vi "Decimate Linear XY.vi"(6 "Width":u32, 8 "error in (no error)":errorcluster, 9 "Xmin":dbl, 10 "Xmax":dbl, 11 "Data to Decimate":cluster{"X":dbl[], "Y":dbl[]}[](array[cluster])) -> (0 "error out":errorcluster, 3 "Decimated Data":cluster{"X":dbl[], "Y":dbl[]}[](array[cluster]))   [LabVIEW 2022 SP3, in "Decimation.lvlib"]
doc: "Decimate XY array to optimize the density of points per pixel to 2 : Min & Max per pixel."
uses:
  Decimation.lvlib
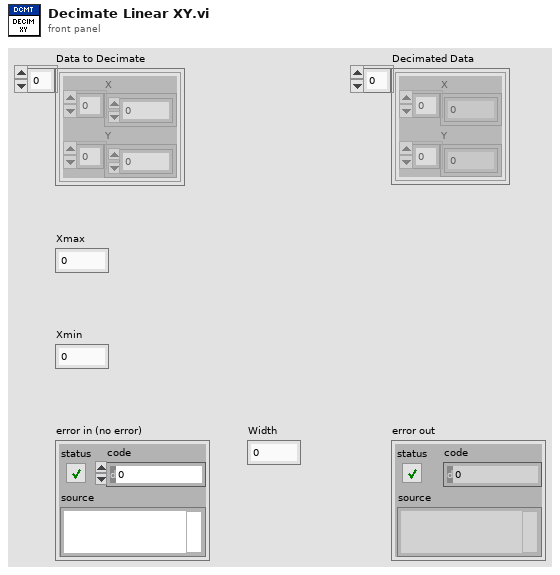
[diagram p1: front panel]
types:
  T1 = cluster{"Decimated Data":dbl[], "Decimated Data":dbl[]}
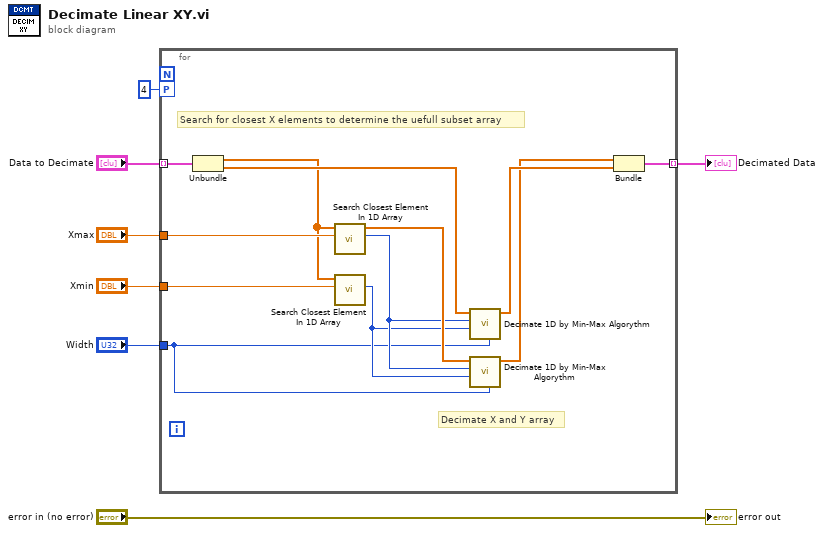
[diagram p0: block diagram]
diagram:
  n1 = for {
    tunnel: "Data to Decimate" -> [w18] mode=indexing
    tunnel: "Xmin" -> [w17]
    tunnel: "Xmax" -> [w16]
    tunnel: [w15] -> w3 mode=indexing
    workers-P: 4 -> [_]
    tunnel: "Width" -> [w10]
    # "Decimate X and Y array"
    # "Search for closest X elements to determine the uefull subset array"
    n2 = Unbundle(w18) -> ("X"=w13:dbl[], "Y"=w14:dbl[])
    n3 = call "Search Closest Element In 1D Array.vi"("Desired element"=w16, "1D Array"=w13) -> ("Closest Index"=w12:i32)  [unwired: 8 in, 1 out]
    n4 = call "Search Closest Element In 1D Array.vi"("Desired element"=w17, "1D Array"=w13) -> ("Closest Index"=w11:i32)  [unwired: 8 in, 1 out]
    n5 = call "Decimate 1D by Min-Max Algorythm.vi"("Width"=w10, "Min Index"=w11, "Max Index"=w12, "Data To Decimate"=w14) -> ("Decimated Data"=w9:dbl[])  [unwired: 6 in, 1 out]
    n6 = call "Decimate 1D by Min-Max Algorythm.vi"("Width"=w10, "Min Index"=w11, "Max Index"=w12, "Data To Decimate"=w13) -> ("Decimated Data"=w8:dbl[])  [unwired: 6 in, 1 out]
    n7 = Bundle("Decimated Data"=w8, "Decimated Data"=w9) -> (w15:T1)  [unwired: 1 in]
  }
  "Decimated Data" <- w3
  "error out" <- "error in (no error)"
